vi "Collect Data.vi"(8 "rate":dbl=1000.0 format="%#_13g", 11 "sample time":i32=1000) -> (3 "Waveform":waveform(dbl))   [LabVIEW 2018]
uses:
  <vilib>/DAQmx/read.llb/DAQmx Read (Analog Wfm 1Chan NSamp).vi
  <vilib>/DAQmx/create/channels.llb/DAQmx Create Channel (AI-Voltage-Basic).vi
  <vilib>/DAQmx/configure/timing.llb/DAQmx Timing (Sample Clock).vi
  <vilib>/DAQmx/miscellaneous.llb/DAQmx Fill In Error Info.vi
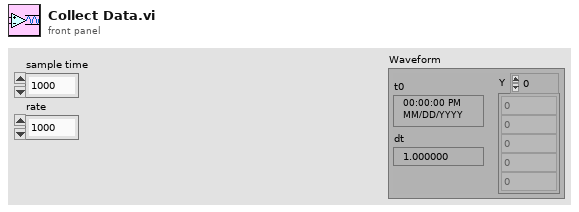
[diagram p1: front panel]
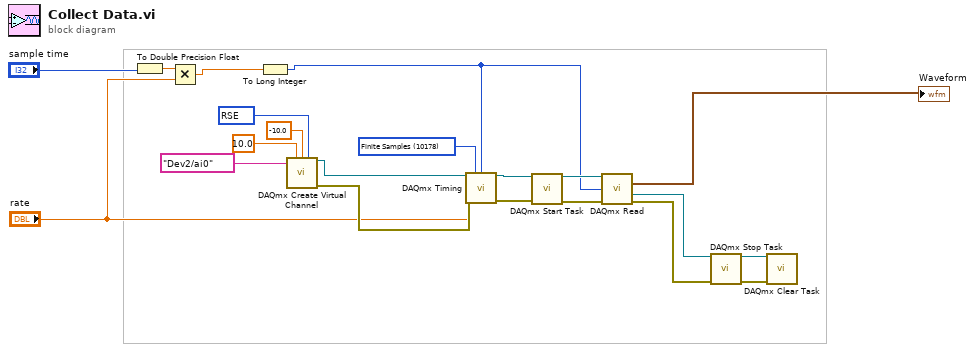
[diagram p0: block diagram]
diagram:
  w8 = 10178 items=["Finite Samples"=10178, "Continuous Samples"=10123, "Hardware Timed Single Point"=12522] ("sample mode")
  w15 = 10083 items=["default"=-1, "RSE"=10083, "NRSE"=10078, "Differential"=10106, "Pseudodifferential"=12529] ("input terminal configuration")
  n1 = To Double Precision Float(number="sample time") -> (double precision float=w3:dbl)
  n2 = Multiply(x=w3, y="rate") -> (x*y=w4:dbl)
  n3 = To Long Integer(number=w4) -> (32bit integer=w1:i32)
  n4 = call-poly <vilib>:"DAQmx Create Virtual Channel.vi"("maximum value"=10.0, "minimum value"=-10.0, "input terminal configuration"=w15, "physical channels"=tag "Dev2/ai0") -> ("task out"=w21:refnum<k21>, "error out"=w12:errorcluster)  [unwired: 10 in]
  n5 = call-poly <vilib>:"DAQmx Timing.vi"("task/channels in"=w21, "sample mode"=w8, "samples per channel"=w1, "rate"="rate", "error in"=w12) -> ("task out"=w20:refnum<k21>, "error out"=w13:errorcluster)  [unwired: 9 in]
  n6 = call <vilib>:"DAQmx Start Task.vi"("task/channels in"=w20, "error in"=w13) -> ("task out"=w19:refnum<k21>, "error out"=w11:errorcluster)  [unwired: 12 in]
  n7 = call-poly <vilib>:"DAQmx Read.vi"("task/channels in"=w19, "number of samples per channel"=w1, "error in"=w11) -> ("task out"=w18:refnum<k21>, "data"=→"Waveform":waveform(dbl), "error out"=w7:errorcluster)  [unwired: 10 in]
  n8 = call <vilib>:"DAQmx Stop Task.vi"("task/channels in"=w18, "error in"=w7) -> ("task out"=w14:refnum<k21>, "error out"=w10:errorcluster)  [unwired: 12 in]
  n9 = call <vilib>:"DAQmx Clear Task.vi"("task in"=w14, "error in"=w10) -> ()  [unwired: 13 in, 1 out]
